vi "Get SMO Public API.vi"(8 "error in (no error)":errorcluster, 11 "Inst.Transport in":refnum<class "Inst.Transport.lvclass">) -> (0 "error out":errorcluster, 2 "Commands":string[](array[string]), 3 "Inst.Transport out":refnum<class "Inst.Transport.lvclass">)   [LabVIEW 2019, in "Inst.Transport.lvclass"]
uses:
  Inst.Transport.lvclass
  <userlib>/LevyLab/Instrument Framework/Instrument Types/SCPI/Instrument.SCPI.lvclass
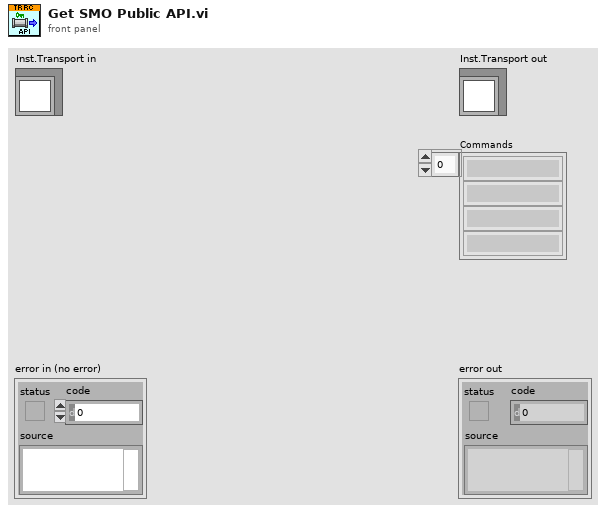
[diagram p1: front panel]
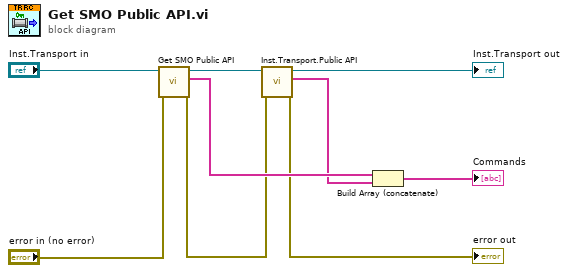
[diagram p0: block diagram]
diagram:
  n1 = call-parent "Get SMO Public API.vi"("error in (no error)"="error in (no error)", "Instrument in"="Inst.Transport in") -> ("error out"=w3:errorcluster, "commands"=w8:string[], "Instrument out"=w4:refnum<class "Inst.Transport.lvclass">)  [unwired: 7 in]
  n2 = call "Inst.Transport.Public API.vi"("error in (no error)"=w3, "Inst.Transport in"=w4) -> ("error out"=→"error out":errorcluster, "commands (this level)"=w5:string[], "Inst.Transport out"=→"Inst.Transport out":refnum<class "Inst.Transport.lvclass">)  [unwired: 7 in]
  n3 = Build Array (concatenate)(w8, w5) -> (→"Commands":string[])
